vi "Demosaic Image.vi"(8 "error in (no error)":errorcluster, 9 "Color Filter Array Phase":i32(ring) items=["BayerRed", "BayerBlue", "BayerGreenLeftOfRed", "BayerGreenLeftOfBlue"], 10 "ImageData":refnum<k24>, 11 "Demosaicker reference in":refnum<k24>) -> (0 "error out":errorcluster, 2 "Demosaicked Data":u16[](array[numeric]), 3 "Demosaicker out":refnum<k24>)   [LabVIEW 2015]
uses:
  C:/code/Host/Installer/Scientific Camera Interfaces/LabVIEW/64_bit/Library_X64/Thorlabs.TSI.Demosaicker.dll
  code/Host/Installer/Scientific Camera Interfaces/LabVIEW/64_bit/Library_X64/Thorlabs.TSI.Demosaicker.dll
  C:/code/Host/Installer/Scientific Camera Interfaces/LabVIEW/64_bit/Library_X64/Thorlabs.TSI.ImageDataInterfaces.dll
  code/Host/Installer/Scientific Camera Interfaces/LabVIEW/64_bit/Library_X64/Thorlabs.TSI.ImageDataInterfaces.dll
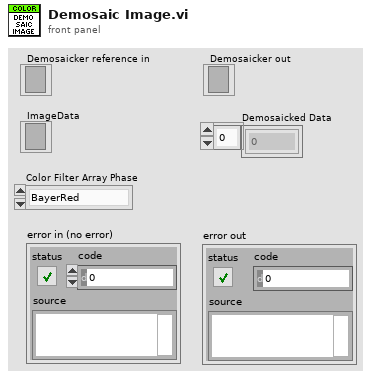
[diagram p1: front panel]
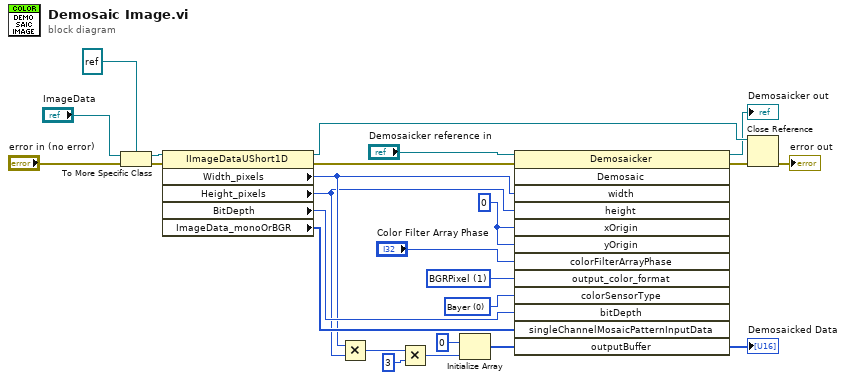
[diagram p0: block diagram]
diagram:
  w15 = 0 items=["Bayer"] ("colorSensorType")
  w16 = 1 items=["BGRPlanar", "BGRPixel", "RGBPixel"] ("output_color_format")
  w18 = 0 ("xOrigin")
  n1 = To More Specific Class(target class=refnum<k24> refnum, reference="ImageData", error in="error in (no error)") -> (specific class reference=w21:refnum<k24>, error out=w20:errorcluster)
  n2 = property class="IImageDataUShort1D"(reference=w21, error in=w20) -> (reference out=w3:refnum<k24>, error out=w19:errorcluster, "Width_pixels"=w11:i32, "Height_pixels"=w10:i32, "BitDepth"=w14:i32, "ImageData_monoOrBGR"=w13:u16[])
  n3 = Multiply(x=w11, y=w10) -> (x*y=w9:i32)
  n4 = Multiply(x=w9, y=3) -> (x*y=w7:i32)
  n5 = Initialize Array(u16 0 ("element"), w7) -> (w6:u16[])
  n6 = invoke class="Demosaicker" method="Demosaic"(reference="Demosaicker reference in", error in=w19, "width"=w11, "height"=w10, "xOrigin"=w18, "yOrigin"=w18, "colorFilterArrayPhase"="Color Filter Array Phase", "output_color_format"=w16, "colorSensorType"=w15, "bitDepth"=w14, "singleChannelMosaicPatternInputData"=w13, "outputBuffer"=w6) -> (reference out=→"Demosaicker out":refnum<k24>, error out=w4:errorcluster, "outputBuffer"=→"Demosaicked Data":u16[])  [unwired: 1 in, 10 out]
  n7 = Close Reference(reference=w3, error in (no error)=w4) -> (error out=→"error out":errorcluster)
